vi "SubPanelControls.vi"() -> ()   [LabVIEW 2016, in "test_ValueSignal.lvlib"]
uses:
  test_ValueSignal.lvlib
  Helper/Helper-SubPanel/Helper-SubPanel.vi
  main/apis/Stimulus/ValueSignalByPathString.vi
  main/apis/Stimulus/ValueSignalByPathArray.vi
  main/apis/Assert/AssertControlValueByPathString.vi
  <vilib>/addons/_JKI Toolkits/Caraya/classes/Assert/Assert Equal Value_Variant.vi
  <vilib>/addons/_JKI Toolkits/Caraya/classes/Assert/Assert.lvclass
  <vilib>/addons/_JKI Toolkits/Caraya/classes/Test/Test.lvclass
panel:
  out "error out":errorcluster
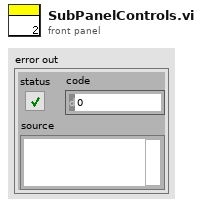
[diagram p1: front panel]
types:
  T1 = typedef "Semaphore RefNum" = refnum<k1>
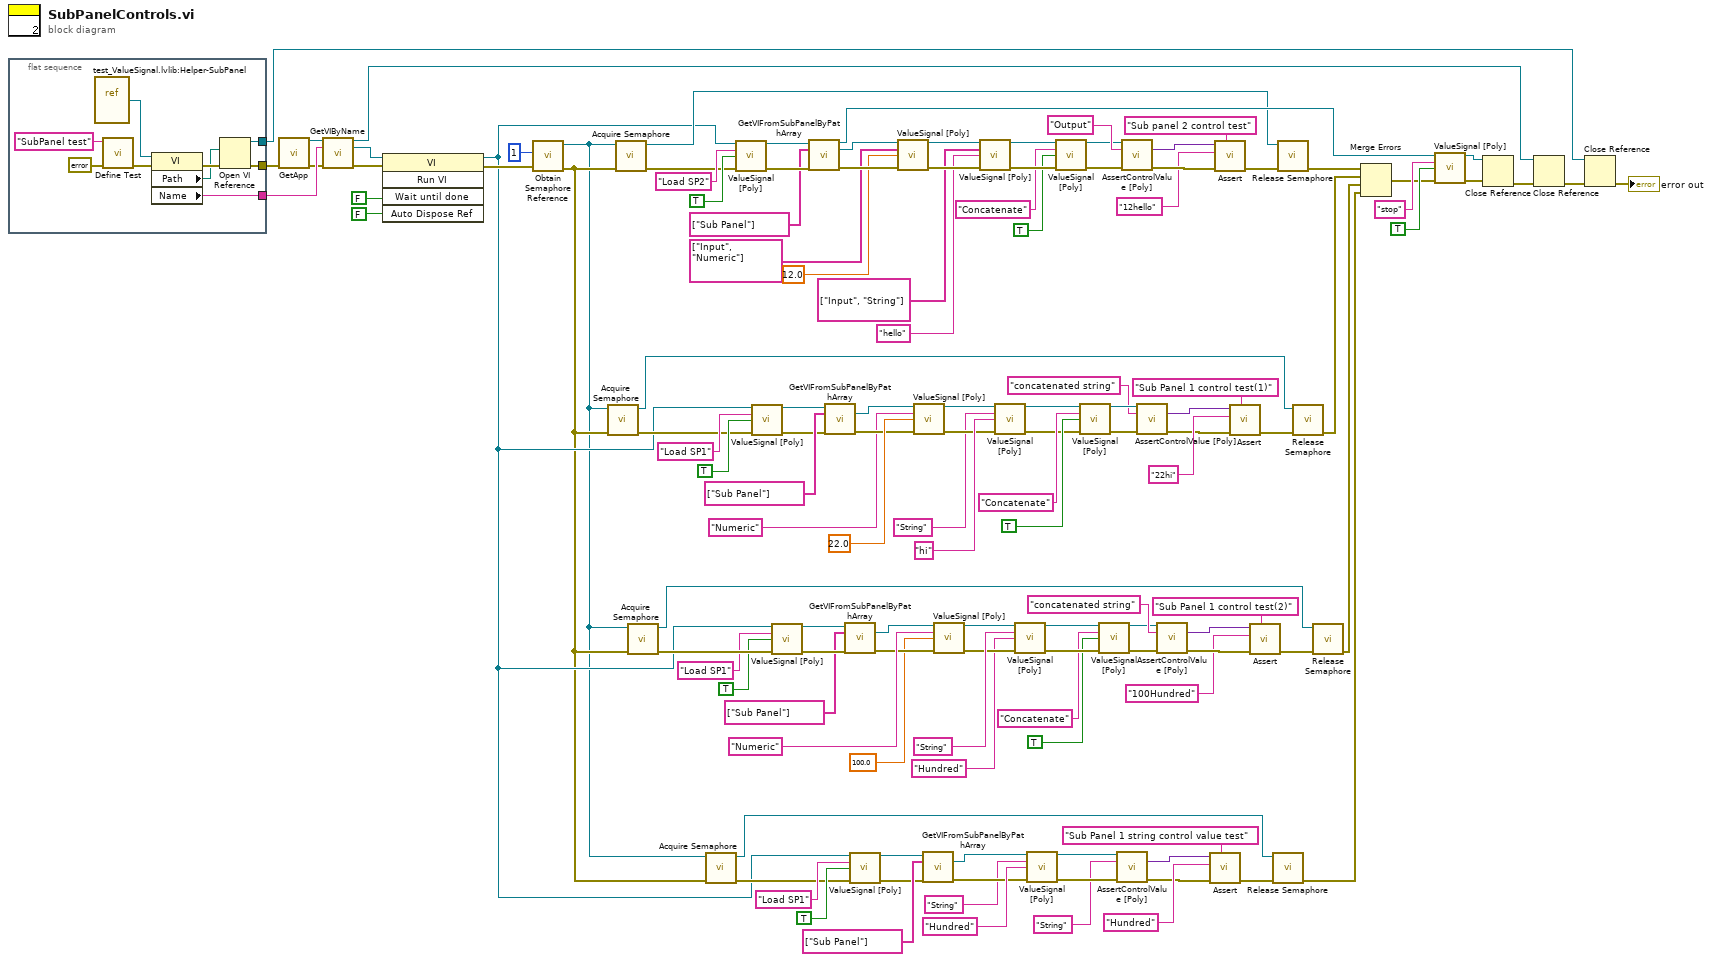
[diagram p0: block diagram]
diagram:
  n1 = flat-sequence {
    tunnel: [w133] -> w125
    tunnel: [w132] -> w127
    tunnel: [w130] -> w124
    frame #0 {
      n2 = vi-ref "test_ValueSignal.lvlib:Helper-SubPanel.vi"() -> (w135:refnum<vi>)
      n3 = call <vilib>:"Define Test.vi"("error in (no error)"=errorcluster {"status"=FALSE, "code"=0, "source"=""}, "Label (VI Title)"="SubPanel test") -> ("error out"=w136:errorcluster)  [unwired: 9 in]
      n4 = property on="Property Node" class="VI"(reference=w135, error in=w136) -> (error out=w134:errorcluster, "Path"=w131:path, "Name"=w130:string)  [unwired: 1 out]
      n5 = Open VI Reference(vi path=w131, error in (no error)=w134) -> (vi reference=w132:refnum<vi>, error out=w133:errorcluster)  [unwired: 4 in]
    }
  }
  n6 = call "GetApp.vi"("error in (no error)"=w125) -> ("Application Ref"=w126:refnum<vi>, "error out"=w123:errorcluster)  [unwired: 13 in]
  n7 = call "GetVIByName.vi"("Application Ref in"=w126, "VI Name"=w124, "error in (no error)"=w123) -> ("Application Ref out"=w121:refnum<vi>, "VI Reference"=w115:refnum<vi>, "error out"=w107:errorcluster)  [unwired: 10 in]
  n8 = invoke on="Invoke Node" class="VI" method="Run VI"(reference=w115, error in=w107, "Wait until done"=FALSE ("Wait Until Done"), "Auto Dispose Ref"=FALSE ("Auto Dispose Reference")) -> (reference out=w4:refnum<vi>, error out=w116:errorcluster)  [unwired: 1 in, 3 out]
  n9 = call <vilib>:"Obtain Semaphore Reference.vi"("error in (no error)"=w116, "size (1)"=1) -> ("error out"=w3:errorcluster, "semaphore"=w2:T1)  [unwired: 3 in, 1 out]
  n10 = call <vilib>:"Acquire Semaphore.vi"("error in (no error)"=w3, "semaphore"=w2) -> ("error out"=w80:errorcluster, "semaphore out"=w79:T1)  [unwired: 3 in, 1 out]
  n11 = call <vilib>:"Acquire Semaphore.vi"("error in (no error)"=w3, "semaphore"=w2) -> ("error out"=w53:errorcluster, "semaphore out"=w52:T1)  [unwired: 3 in, 1 out]
  n12 = call <vilib>:"Acquire Semaphore.vi"("error in (no error)"=w3, "semaphore"=w2) -> ("error out"=w50:errorcluster, "semaphore out"=w51:T1)  [unwired: 3 in, 1 out]
  n13 = call <vilib>:"Acquire Semaphore.vi"("error in (no error)"=w3, "semaphore"=w2) -> ("error out"=w6:errorcluster, "semaphore out"=w5:T1)  [unwired: 3 in, 1 out]
  n14 = call-poly "ValueSignal [Poly].vi"("VI Reference In"=w4, "Control Name"="Load SP2" ("Class Name"), "Value (Signaling)"=TRUE, "error in"=w53) -> ("VI Reference Out"=w72:refnum<vi>, "error out"=w73:errorcluster)  [unwired: 10 in]
  n15 = call-poly "ValueSignal [Poly].vi"("VI Reference In"=w4, "Control Name"="Load SP1" ("Class Name"), "Value (Signaling)"=TRUE, "error in"=w80) -> ("VI Reference Out"=w89:refnum<vi>, "error out"=w88:errorcluster)  [unwired: 10 in]
  n16 = call-poly "ValueSignal [Poly].vi"("VI Reference In"=w4, "Control Name"="Load SP1" ("Class Name"), "Value (Signaling)"=TRUE, "error in"=w50) -> ("VI Reference Out"=w41:refnum<vi>, "error out"=w42:errorcluster)  [unwired: 10 in]
  n17 = call "GetVIFromSubPanelByPathArray.vi"("VI Reference in"=w72, "SubPanel Path"=string[] ["Sub Panel"], "error in (no error)"=w73) -> ("VI Reference out"=w109:refnum<vi>, "SubPanel VI Reference"=w69:refnum<vi>, "error out"=w70:errorcluster)  [unwired: 10 in]
  n18 = call "GetVIFromSubPanelByPathArray.vi"("VI Reference in"=w89, "SubPanel Path"=string[] ["Sub Panel"], "error in (no error)"=w88) -> ("SubPanel VI Reference"=w92:refnum<vi>, "error out"=w91:errorcluster)  [unwired: 10 in, 1 out]
  n19 = call "GetVIFromSubPanelByPathArray.vi"("VI Reference in"=w41, "SubPanel Path"=string[] ["Sub Panel"], "error in (no error)"=w42) -> ("SubPanel VI Reference"=w38:refnum<vi>, "error out"=w39:errorcluster)  [unwired: 10 in, 1 out]
  n20 = call-poly "ValueSignal [Poly].vi"("VI Reference In"=w4, "Control Name"="Load SP1" ("Class Name"), "Value (Signaling)"=TRUE, "error in"=w6) -> ("VI Reference Out"=w14:refnum<vi>, "error out"=w13:errorcluster)  [unwired: 10 in]
  n21 = call-poly "ValueSignal [Poly].vi"("VI Reference In"=w69, "Control Path"=string[] ["Input", "Numeric"], "Value (Signaling)"=12.0, "error in"=w70) -> ("VI Reference Out"=w64:refnum<vi>, "error out"=w65:errorcluster)  [unwired: 10 in]
  n22 = call-poly "ValueSignal [Poly].vi"("VI Reference In"=w92, "Control Name"="Numeric", "Value (Signaling)"=22.0, "error in"=w91) -> ("VI Reference Out"=w96:refnum<vi>, "error out"=w95:errorcluster)  [unwired: 10 in]
  n23 = call "GetVIFromSubPanelByPathArray.vi"("VI Reference in"=w14, "SubPanel Path"=string[] ["Sub Panel"], "error in (no error)"=w13) -> ("SubPanel VI Reference"=w17:refnum<vi>, "error out"=w16:errorcluster)  [unwired: 10 in, 1 out]
  n24 = call-poly "ValueSignal [Poly].vi"("VI Reference In"=w38, "Control Name"="Numeric", "Value (Signaling)"=100.0, "error in"=w39) -> ("VI Reference Out"=w34:refnum<vi>, "error out"=w35:errorcluster)  [unwired: 10 in]
  n25 = call-poly "ValueSignal [Poly].vi"("VI Reference In"=w64, "Control Path"=string[] ["Input", "String"], "Value (Signaling)"="hello" ("Control Name"), "error in"=w65) -> ("VI Reference Out"=w58:refnum<vi>, "error out"=w60:errorcluster)  [unwired: 10 in]
  n26 = call-poly "ValueSignal [Poly].vi"("VI Reference In"=w96, "Control Name"="String", "Value (Signaling)"="hi" ("Control Name"), "error in"=w95) -> ("VI Reference Out"=w101:refnum<vi>, "error out"=w99:errorcluster)  [unwired: 10 in]
  n27 = call-poly "ValueSignal [Poly].vi"("VI Reference In"=w34, "Control Name"="String", "Value (Signaling)"="Hundred" ("Control Name"), "error in"=w35) -> ("VI Reference Out"=w29:refnum<vi>, "error out"=w31:errorcluster)  [unwired: 10 in]
  n28 = call-poly "ValueSignal [Poly].vi"("VI Reference In"=w17, "Control Name"="String", "Value (Signaling)"="Hundred" ("Control Name"), "error in"=w16) -> ("VI Reference Out"=w22:refnum<vi>, "error out"=w21:errorcluster)  [unwired: 10 in]
  n29 = call-poly "ValueSignal [Poly].vi"("VI Reference In"=w58, "Control Name"="Concatenate", "Value (Signaling)"=TRUE, "error in"=w60) -> ("VI Reference Out"=w57:refnum<vi>, "error out"=w59:errorcluster)  [unwired: 10 in]
  n30 = call-poly "ValueSignal [Poly].vi"("VI Reference In"=w101, "Control Name"="Concatenate", "Value (Signaling)"=TRUE, "error in"=w99) -> ("VI Reference Out"=w102:refnum<vi>, "error out"=w100:errorcluster)  [unwired: 10 in]
  n31 = call-poly "ValueSignal [Poly].vi"("VI Reference In"=w29, "Control Name"="Concatenate", "Value (Signaling)"=TRUE, "error in"=w31) -> ("VI Reference Out"=w28:refnum<vi>, "error out"=w30:errorcluster)  [unwired: 10 in]
  n32 = call-poly "AssertControlValue [Poly].vi"("VI Reference In"=w22, "Control Name"="String", "error in"=w21) -> ("Value"=w11:variant, "error out"=w10:errorcluster)  [unwired: 10 in, 1 out]
  n33 = call-poly "AssertControlValue [Poly].vi"("VI Reference In"=w57, "Control Name"="Output", "error in"=w59) -> ("Value"=w75:variant, "error out"=w76:errorcluster)  [unwired: 10 in, 1 out]
  n34 = call-poly "AssertControlValue [Poly].vi"("VI Reference In"=w102, "Control Name"="concatenated string", "error in"=w100) -> ("Value"=w86:variant, "error out"=w85:errorcluster)  [unwired: 10 in, 1 out]
  n35 = call-poly "AssertControlValue [Poly].vi"("VI Reference In"=w28, "Control Name"="concatenated string", "error in"=w30) -> ("Value"=w44:variant, "error out"=w45:errorcluster)  [unwired: 10 in, 1 out]
  n36 = call-poly <vilib>:"Assert.vi"("Label"="Sub Panel 1 string control value test" ("Label (VI Title)"), "error in (no error)"=w10, "Y"="Hundred" ("Control Name"), "X"=w11) -> ("error out"=w23:errorcluster)  [unwired: 7 in]
  n37 = call-poly <vilib>:"Assert.vi"("Label"="Sub panel 2 control test" ("Label (VI Title)"), "error in (no error)"=w76, "Y"="12hello" ("Control Name"), "X"=w75) -> ("error out"=w54:errorcluster)  [unwired: 7 in]
  n38 = call-poly <vilib>:"Assert.vi"("Label"="Sub Panel 1 control test(1)" ("Label (VI Title)"), "error in (no error)"=w85, "Y"="22hi" ("Control Name"), "X"=w86) -> ("error out"=w105:errorcluster)  [unwired: 7 in]
  n39 = call-poly <vilib>:"Assert.vi"("Label"="Sub Panel 1 control test(2)" ("Label (VI Title)"), "error in (no error)"=w45, "Y"="100Hundred" ("Control Name"), "X"=w44) -> ("error out"=w25:errorcluster)  [unwired: 7 in]
  n40 = call <vilib>:"Release Semaphore.vi"("error in (no error)"=w23, "semaphore"=w5) -> ("error out"=w1:errorcluster)  [unwired: 4 in, 1 out]
  n41 = call <vilib>:"Release Semaphore.vi"("error in (no error)"=w54, "semaphore"=w52) -> ("error out"=w114:errorcluster)  [unwired: 4 in, 1 out]
  n42 = call <vilib>:"Release Semaphore.vi"("error in (no error)"=w105, "semaphore"=w79) -> ("error out"=w119:errorcluster)  [unwired: 4 in, 1 out]
  n43 = call <vilib>:"Release Semaphore.vi"("error in (no error)"=w25, "semaphore"=w51) -> ("error out"=w24:errorcluster)  [unwired: 4 in, 1 out]
  n44 = Merge Errors(w114, w119, w24, w1) -> (w111:errorcluster)
  n45 = call-poly "ValueSignal [Poly].vi"("VI Reference In"=w109, "Control Name"="stop" ("Class Name"), "Value (Signaling)"=TRUE, "error in"=w111) -> ("VI Reference Out"=w108:refnum<vi>, "error out"=w110:errorcluster)  [unwired: 10 in]
  n46 = Close Reference(reference=w108, error in (no error)=w110) -> (error out=w120:errorcluster)
  n47 = Close Reference(reference=w121, error in (no error)=w120) -> (error out=w122:errorcluster)
  n48 = Close Reference(reference=w127, error in (no error)=w122) -> (error out=→"error out":errorcluster)
